vi "set cluster to new location.vi"(8 "error in":errorcluster, 11 "Set Cluster":T1) -> (0 "error out":errorcluster, 1 "num pages":i32, 2 "Location Cluster out":T2, 3 "set index":i32)   [LabVIEW 2018]
uses:
  location cluster.ctl
  set location.ctl
  CAEN globals.vi
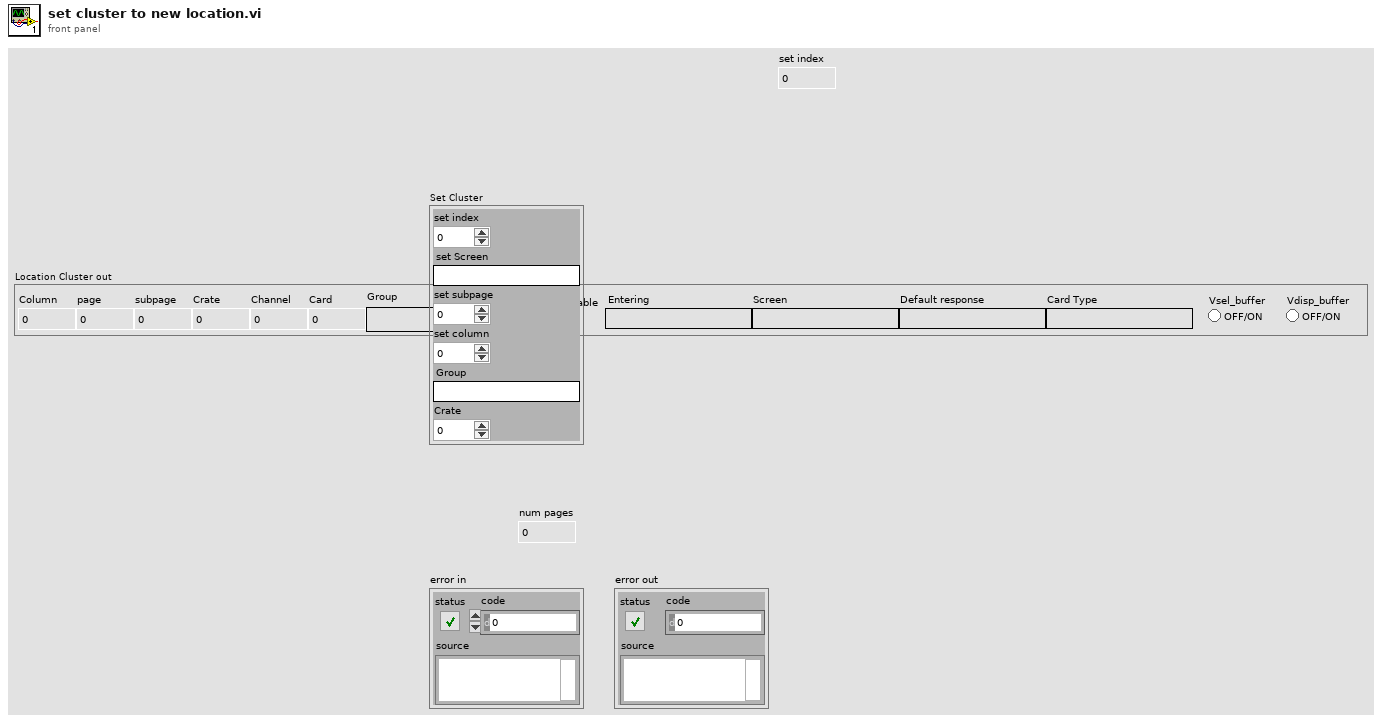
[diagram p1: front panel]
types:
  T1 = typedef "set location.ctl" = cluster{"set index":i32, "set Screen":string, "set subpage":i32, "set column":i32, "Group":string, "Crate":i32}
  T2 = typedef "location cluster.ctl" = cluster{"Column":i32, "Card Type":string, "Channel":i32, "Card":i32, "Default response":string, "Entering":string, "Entering state":bool, "subpage":i32, "page":i32, "Crate":i32, "Screen":string, "Group":string, "Global HV Enable":bool, "Vsel_buffer":bool, "Vdisp_buffer":bool}
  T3 = typedef "channel.ctl" = cluster{" Card.Channel":dbl, "Crate":i32}
  T4 = cluster{"Group Name":string, "Channels in Group":T3[]}[]
  T5 = typedef "crate.ctl" = cluster{"CAENet Address":i32, "Crate Model":string, "Firmware Version":string, "Crate Map":T6[], "Total Channels":i32}
  T6 = typedef "card.ctl" = cluster{"Slot Number":i32, "Card Model":string, "Num Channels":i32, "Polarity":string, "Vmax":dbl, "Imax":dbl, "Revision":string}
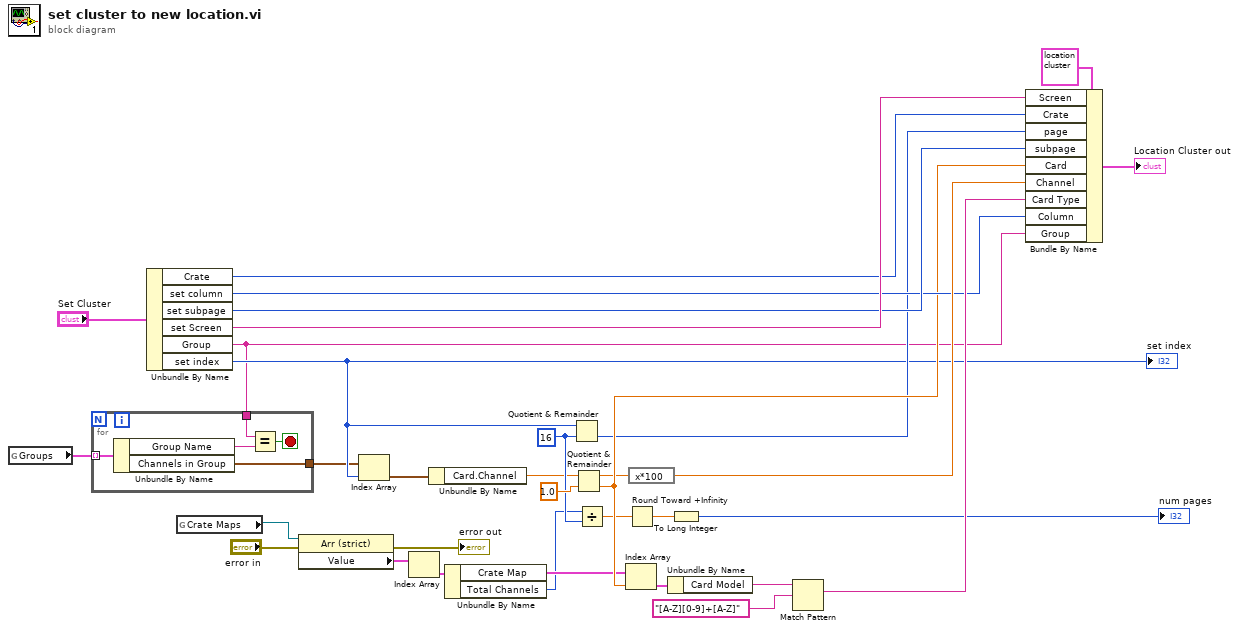
[diagram p0: block diagram]
diagram:
  w11 = 16 ("y")
  n1 = global read "CAEN globals.vi" "Groups"() -> (w17:T4)
  n2 = Unbundle By Name("Set Cluster") -> ("Crate"=w5:i32, "set column"=w29:i32, "set subpage"=w30:i32, "set Screen"=w33:string, "Group"=w20:string, "set index"=w21:i32)
  "set index" <- w21
  n3 = for {
    tunnel: w17 -> [w38] mode=indexing
    tunnel: [w36] -> w12
    tunnel: w20 -> [w34]
    stop <- w37 stop-if-true
    n4 = Unbundle By Name(w38) -> ("Group Name"=w35:string, "Channels in Group"=w36:T3[])
    n5 = Equal?(x=w34, y=w35) -> (x = y?=w37:bool)
  }
  n6 = global read "CAEN globals.vi" "Crate Maps"() -> (w16:refnum<vi>)
  n7 = property class="Arr (strict)"(reference=w16, error in="error in") -> (error out=→"error out":errorcluster, "Value"=w15:T5[])  [unwired: 1 out]
  n8 = Index Array(array=w12, index=w21) -> (element=w4:T3)
  n9 = Index Array(array=w15) -> (element=w2:T5)  [unwired: 1 in]
  n10 = Unbundle By Name(w4) -> ("Card.Channel"=w3:dbl)
  n11 = Unbundle By Name(w2) -> ("Crate Map"=w14:T6[], "Total Channels"=w1:i32)
  n12 = Quotient & Remainder(x=w21, y=w11) -> (floor(x/y)=w22:i32)  [unwired: 1 out]
  n13 = Quotient & Remainder(x=w3, y=1.0) -> (x-y*floor(x/y)=w19:dbl, floor(x/y)=w24:dbl)
  n14 = Divide(x=w1, y=w11) -> (x/y=w10:dbl)
  n15 = Index Array(array=w14, index=w24) -> (element=w13:T6)
  n16 = Round Toward +Infinity(x=w10) -> (ceil(x): smallest int >= x=w7:dbl)
  n17 = expression code="x*100"(w19) -> (w32:dbl)
  n18 = Unbundle By Name(w13) -> ("Card Model"=w8:string)
  n19 = To Long Integer(number=w7) -> (32bit integer=→"num pages":i32)
  n20 = Match Pattern(string=w8, regular expression="[A-Z][0-9]+[A-Z]") -> (match substring=w31:string)  [unwired: 1 in, 3 out]
  n21 = Bundle By Name(cluster=T2 {"Column"=0, "Card Type"="", "Channel"=0, "Card"=0, "Default response"="", "Entering"="", "Entering state"=FALSE, "subpage"=0, "page"=0, "Crate"=0, "Screen"="", "Group"="", "Global HV Enable"=FALSE, "Vsel_buffer"=FALSE, "Vdisp_buffer"=FALSE} ("Location Cluster out"), "Screen"=w33, "Crate"=w5, "page"=w22, "subpage"=w30, "Card"=w24, "Channel"=w32, "Card Type"=w31, "Column"=w29, "Group"=w20) -> (→"Location Cluster out":T2)
